vi "Conversao_valores_UCM.0300_ENTRADA.vi"(8 "Instrumentos":T1, 11 "UCM.004.EEL.0300_ENTRADA(Controle)":T3) -> (3 "UCM.004.EEL.0300_ENTRADA(Indicador)":T3)   [LabVIEW 2019]
uses:
  padrao_UCM.004.EEL.0300_ENTRADA.ctl
  padrao_array_cluster_calibracao.ctl
  <vilib>/Utility/Data Type/NI_Data Type.lvlib
panel:
  out "ANALOGICO_entrada":T2
  in  "ANALOGICO_saida":T2
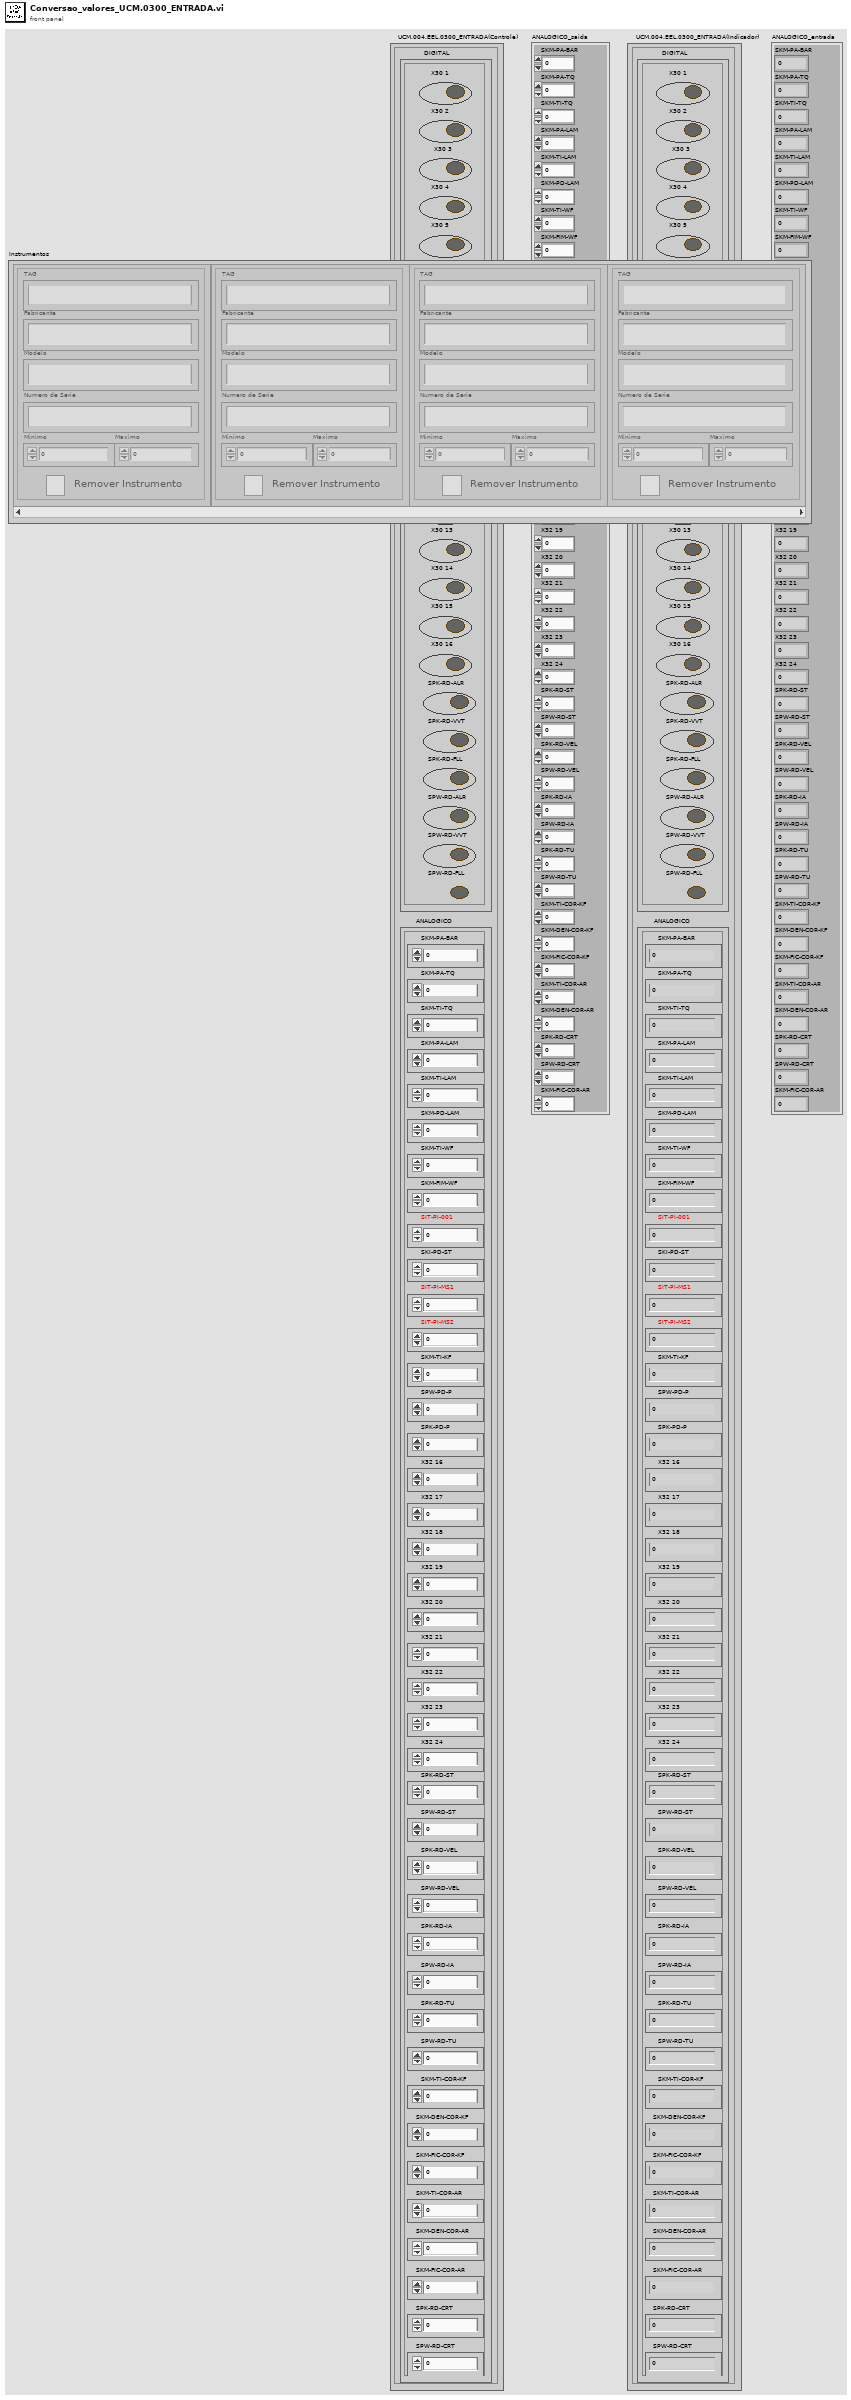
[diagram p1: front panel]
types:
  T1 = typedef "padrao_array_cluster_calibracao.ctl" = cluster{"TAG":string, "Minimo":dbl, "Fabricante":string, "Maximo":dbl, "remover_dipositvo":bool, "Modelo":string, "Numero de Serie":string}[]
  T2 = cluster{"SKM-PA-BAR":i16, "SKM-PA-TQ":i16, "SKM-TI-TQ":i16, "SKM-PA-LAM":i16, "SKM-TI-LAM":i16, "SKM-PD-LAM":i16, "SKM-TI-WF":i16, "SKM-FIM-WF":i16, "SIT-PI-001":i16, "SKI-PD-ST":i16, "SIT-PI-MS1":i16, "SIT-PI-MS2":i16, "SKM-TI-KF":i16, "SPW-PD-P":i16, "SPK-PD-P":i16, "X32 16 ":i16, "X32 17":i16, "X32 18":i16, "X32 19":i16, "X32 20":i16, "X32 21":i16, "X32 22":i16, "X32 23":i16, "X32 24":i16, "SPK-RD-ST":i16, "SPW-RD-ST":i16, "SPK-RD-VEL":i16, "SPW-RD-VEL":i16, "SPK-RD-IA":i16, "SPW-RD-IA":i16, "SPK-RD-TU":i16, "SPW-RD-TU":i16, "SKM-TI-COR-KF":dbl, "SKM-DEN-COR-KF":dbl, "SKM-FIC-COR-KF":dbl, "SKM-TI-COR-AR":dbl, "SKM-DEN-COR-AR":dbl, "SPK-RD-CRT":dbl, "SPW-RD-CRT":dbl, "SKM-FIC-COR-AR":dbl}
  T3 = typedef "padrao_UCM.004.EEL.0300_ENTRADA.ctl" = cluster{"DIGITAL":cluster{"X30 1":bool, "X30 2":bool, "X30 3":bool, "X30 4":bool, "X30 5":bool, "X30 6":bool, "X30 7":bool, "X30 8":bool, "X30 9":bool, "X30 10":bool, "X30 11":bool, "X30 12":bool, "X30 13":bool, "X30 14":bool, "X30 15":bool, "X30 16":bool, "SPK-RD-ALR":bool, "SPK-RD-VVT":bool, "SPK-RD-FLL":bool, "SPW-RD-ALR":bool, "SPW-RD-VVT":bool, "SPW-RD-FLL":bool}, "ANALOGICO":cluster{"SKM-PA-BAR":i16, "SKM-PA-TQ":i16, "SKM-TI-TQ":i16, "SKM-PA-LAM":i16, "SKM-TI-LAM":i16, "SKM-PD-LAM":i16, "SKM-TI-WF":i16, "SKM-FIM-WF":i16, "SIT-PI-001":i16, "SKI-PD-ST":i16, "SIT-PI-MS1":i16, "SIT-PI-MS2":i16, "SKM-TI-KF":i16, "SPW-PD-P":i16, "SPK-PD-P":i16, "X32 16 ":i16, "X32 17":i16, "X32 18":i16, "X32 19":i16, "X32 20":i16, "X32 21":i16, "X32 22":i16, "X32 23":i16, "X32 24":i16, "SPK-RD-ST":i32, "SPW-RD-ST":i32, "SPK-RD-VEL":i32, "SPW-RD-VEL":i32, "SPK-RD-IA":i32, "SPW-RD-IA":i32, "SPK-RD-TU":i32, "SPW-RD-TU":i32, "SKM-TI-COR-KF":dbl, "SKM-DEN-COR-KF":dbl, "SKM-FIC-COR-KF":dbl, "SKM-TI-COR-AR":dbl, "SKM-DEN-COR-AR":dbl, "SPK-RD-CRT":dbl, "SPW-RD-CRT":dbl, "SKM-FIC-COR-AR":dbl}}
  T4 = cluster{"SKM-PA-BAR":i16, "SKM-PA-TQ":i16, "SKM-TI-TQ":i16, "SKM-PA-LAM":i16, "SKM-TI-LAM":i16, "SKM-PD-LAM":i16, "SKM-TI-WF":i16, "SKM-FIM-WF":i16, "SIT-PI-001":i16, "SKI-PD-ST":i16, "SIT-PI-MS1":i16, "SIT-PI-MS2":i16, "SKM-TI-KF":i16, "SPW-PD-P":i16, "SPK-PD-P":i16, "X32 16 ":i16, "X32 17":i16, "X32 18":i16, "X32 19":i16, "X32 20":i16, "X32 21":i16, "X32 22":i16, "X32 23":i16, "X32 24":i16, "SPK-RD-ST":i32, "SPW-RD-ST":i32, "SPK-RD-VEL":i32, "SPW-RD-VEL":i32, "SPK-RD-IA":i32, "SPW-RD-IA":i32, "SPK-RD-TU":i32, "SPW-RD-TU":i32, "SKM-TI-COR-KF":dbl, "SKM-DEN-COR-KF":dbl, "SKM-FIC-COR-KF":dbl, "SKM-TI-COR-AR":dbl, "SKM-DEN-COR-AR":dbl, "SPK-RD-CRT":dbl, "SPW-RD-CRT":dbl, "SKM-FIC-COR-AR":dbl}
  T5 = cluster{"TAG":string, "Minimo":dbl, "Fabricante":string, "Maximo":dbl, "remover_dipositvo":bool, "Modelo":string, "Numero de Serie":string}
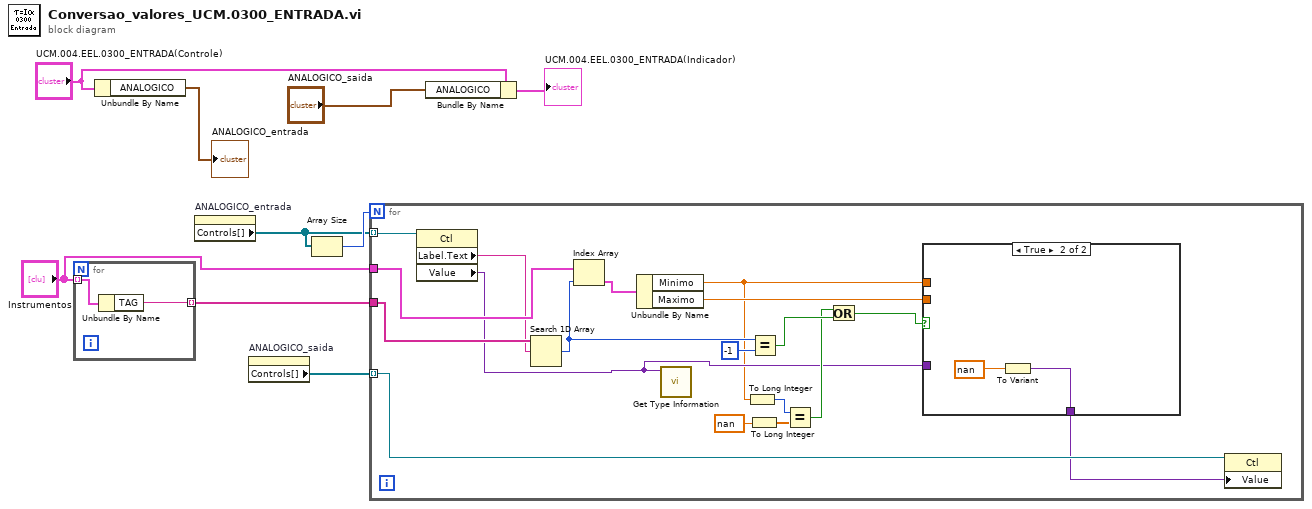
[diagram p0: block diagram]
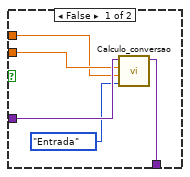
[diagram p2: hidden frame]
diagram:
  n1 = for {
    tunnel: "Instrumentos" -> [w11] mode=indexing
    tunnel: [w10] -> w5 mode=indexing
    n2 = Unbundle By Name(w11) -> ("TAG"=w10:string)
  }
  n3 = Unbundle By Name("UCM.004.EEL.0300_ENTRADA(Controle)") -> ("ANALOGICO"=→"ANALOGICO_entrada":T4)
  n4 = property on="ANALOGICO_entrada" class="Clust (strict)"() -> ("Controls[]"=w2:refnum<vi>[])  [unwired: 2 in, 2 out]
  n5 = property on="ANALOGICO_saida" class="Clust (strict)"() -> ("Controls[]"=w1:refnum<vi>[])  [unwired: 2 in, 2 out]
  n6 = Array Size(array=w2) -> (size(s)=w3:i32)
  n7 = for {
    N: w3 -> [_]
    tunnel: w2 -> [w29] mode=indexing
    tunnel: w1 -> [w25] mode=indexing
    tunnel: w5 -> [w28]
    tunnel: "Instrumentos" -> [w27]
    n8 = property class="Ctl"(reference=w29) -> ("Label.Text"=w24:string, "Value"=w16:variant)  [unwired: 1 in, 2 out]
    n9 = Search 1D Array(1D array=w28, element=w24) -> (index of element=w23:i32)  [unwired: 1 in]
    n10 = Index Array(array=w27, index=w23) -> (element=w26:T5)
    n11 = Unbundle By Name(w26) -> ("Minimo"=w12:dbl, "Maximo"=w13:dbl)
    n12 = call <vilib>:"Get Type Information.vi"("variant"=w16) -> ()  [unwired: 6 in, 5 out]
    n13 = To Long Integer(number=w12) -> (32bit integer=w19:i32)
    n14 = To Long Integer(number=nan) -> (32bit integer=w18:i32)
    n15 = Equal?(x=w23, y=-1) -> (x = y?=w21:bool)
    n16 = Equal?(x=w19, y=w18) -> (x = y?=w17:bool)
    n17 = Or(x=w17, y=w21) -> (x .or. y?=w14:bool)
    n18 = case shown="True" w14 {
      tunnel: w16 -> [w34 _]
      tunnel: [w33 w35] -> w15
      tunnel: w13 -> [w32 _]
      tunnel: w12 -> [w31 _]
      frame False {
        n19 = call "Calculo_conversao.vi"("Tipo"=enum16{"Saida", "Entrada"}."Entrada", "Min"=w31, "Max"=w32, "Value"=w34) -> ("Value 2"=w33:variant)  [unwired: 7 in]
      }
      frame True {
        n20 = To Variant(anything=nan) -> (Variant=w35:variant)
      }
    }
    n21 = property class="Ctl"(reference=w25, "Value"=w15) -> ()  [unwired: 1 in, 2 out]
  }
  n22 = Bundle By Name(cluster="UCM.004.EEL.0300_ENTRADA(Controle)", "ANALOGICO"="ANALOGICO_saida") -> (→"UCM.004.EEL.0300_ENTRADA(Indicador)":T3)
